vi "Go To Position.vi"(8 "error in (no error)":errorcluster, 9 "Target Position":T2, 10 "My Position":T2) -> (0 "error out":errorcluster, 1 "Arrived?":bool, 2 "Direction":T1)   [LabVIEW 2015, in "Common.lvlib"]
uses:
  Common.lvlib
  Position.ctl
  Type Defs/Direction Enum.ctl
  SubVIs/Read-Only Globals.vi
  SubVIs/Globals (private).vi
  Type Defs/SB Type Defs.lvlib
  Square/Square.lvclass
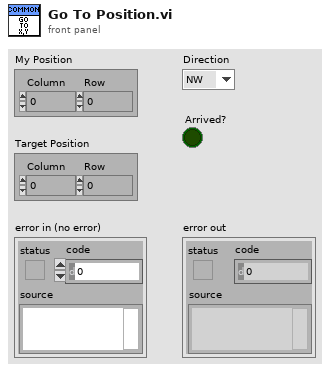
[diagram p1: front panel]
types:
  T1 = typedef "SB Type Defs.lvlib/Direction Enum.ctl" = enum16{"NW", "N", "NE", "E", "SE", "S", "SW", "W"}
  T2 = typedef "Common.lvlib/Position.ctl" = cluster{"Column":i32, "Row":i32}
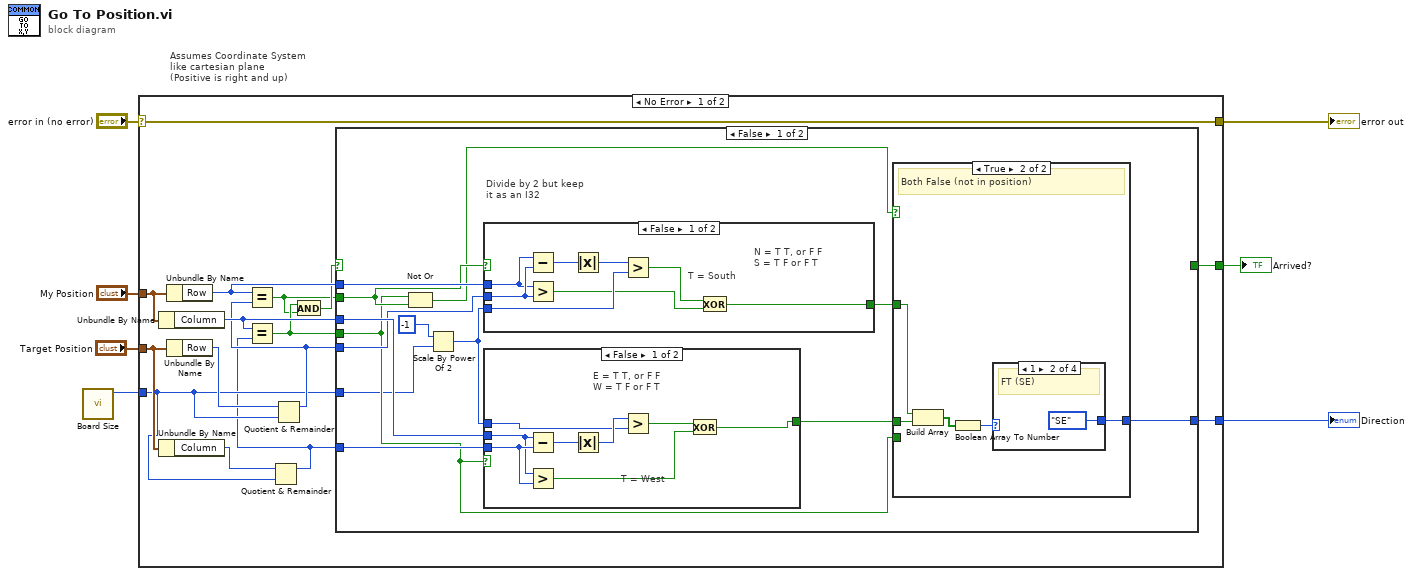
[diagram p0: block diagram]
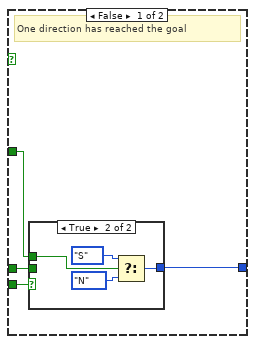
[diagram p2: hidden frame]
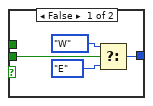
[diagram p3: hidden frame]
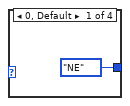
[diagram p4: hidden frame]
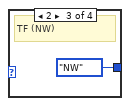
[diagram p5: hidden frame]
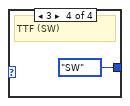
[diagram p6: hidden frame]
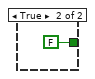
[diagram p7: hidden frame]
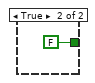
[diagram p8: hidden frame]
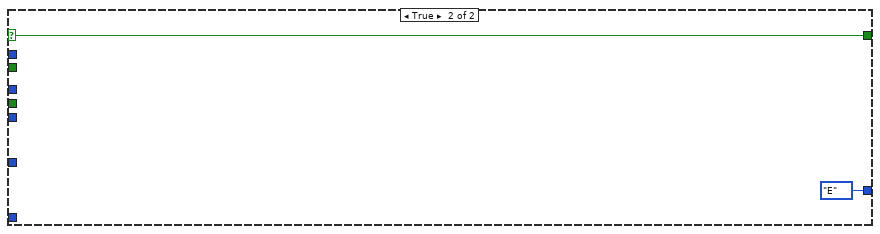
[diagram p9: hidden frame]
diagram:
  # "Assumes Coordinate System\nlike cartesian plane\n(Positive is right and up)"
  n1 = call "Board Size.vi"() -> ("Board Size"=w1:i32)  [unwired: 11 in]
  n2 = case shown="No Error" "error in (no error)" {
    selector: "error in (no error)" -> [w22 w77]
    tunnel: [w22 w77] -> w6
    tunnel: "Target Position" -> [w20 _]
    tunnel: "My Position" -> [w21 _]
    tunnel: [w16 _] -> w3
    tunnel: [w14 _] -> w2
    tunnel: w1 -> [w9 _]
    frame No Error {
      n3 = Unbundle By Name(w21) -> ("Column"=w19:i32)
      n4 = Unbundle By Name(w20) -> ("Column"=w10:i32)
      n5 = Unbundle By Name(w21) -> ("Row"=w18:i32)
      n6 = Unbundle By Name(w20) -> ("Row"=w12:i32)
      n7 = Quotient & Remainder(x=w10, y=w9) -> (x-y*floor(x/y)=w8:i32)  [unwired: 1 out]
      n8 = Equal?(x=w19, y=w8) -> (x = y?=w17:bool)
      n9 = Quotient & Remainder(x=w12, y=w9) -> (x-y*floor(x/y)=w11:i32)  [unwired: 1 out]
      n10 = Equal?(x=w18, y=w11) -> (x = y?=w13:bool)
      n11 = And(x=w17, y=w13) -> (x .and. y?=w15:bool)
      n12 = case shown="False" w15 {
        selector: w15 -> [_ w75]
        tunnel: w8 -> [w34 _]
        tunnel: w19 -> [w33 _]
        tunnel: w18 -> [w32 _]
        tunnel: w11 -> [w31 _]
        tunnel: w17 -> [w25 _]
        tunnel: [w24 Direction_Enum."E" ("Direction")] -> w16
        tunnel: [_ w75] -> w14
        tunnel: w13 -> [w29 _]
        tunnel: w9 -> [w23 _]
        frame False {
          # "Divide by 2 but keep it as an I32"
          n13 = Not Or(1:w29, 2:w25) -> (0:w28:bool)
          n14 = Scale By Power Of 2(n=i16 -1, x=w23) -> (x*2^n=w30:i32)
          n15 = case shown="False" w29 {
            tunnel: w30 -> [w62 _]
            tunnel: w31 -> [w61 _]
            tunnel: w32 -> [w60 _]
            tunnel: [w57 FALSE] -> w26
            frame False {
              # "T = South"
              # "N = T T, or F F\nS = T F or F T"
              n16 = Subtract(x=w60, y=w61) -> (x-y=w63:i32)
              n17 = Greater?(x=w60, y=w61) -> (0:w58:bool)
              n18 = Absolute Value(x=w63) -> (abs(x)=w64:i32)
              n19 = Greater?(x=w64, y=w62) -> (0:w59:bool)
              n20 = Exclusive Or(1:w58, 2:w59) -> (0:w57:bool)
            }
            frame True {
            }
          }
          n21 = case shown="False" w25 {
            tunnel: w30 -> [w71 _]
            tunnel: w34 -> [w70 _]
            tunnel: w33 -> [w69 _]
            tunnel: [w66 FALSE] -> w27
            frame False {
              # "T = West"
              # "E = T T, or F F\nW = T F or F T"
              n22 = Subtract(x=w69, y=w70) -> (x-y=w72:i32)
              n23 = Greater?(x=w69, y=w70) -> (0:w67:bool)
              n24 = Absolute Value(x=w72) -> (abs(x)=w73:i32)
              n25 = Greater?(x=w73, y=w71) -> (0:w68:bool)
              n26 = Exclusive Or(1:w67, 2:w68) -> (0:w66:bool)
            }
            frame True {
            }
          }
          n27 = case shown="True" w28 {
            tunnel: w27 -> [w38 w52]
            tunnel: w26 -> [w36 w51]
            tunnel: w25 -> [w39 _]
            tunnel: [w37 w48] -> w24
            frame False {
              # "One direction has reached the goal"
              n28 = case shown="True" w39 {
                tunnel: [w40 w44] -> w37
                tunnel: w38 -> [w43 _]
                tunnel: w36 -> [_ w45]
                frame False {
                  n29 = Select(t=Direction_Enum."W" ("Direction"), s=w43, f=Direction_Enum."E" ("Direction")) -> (s? t:f=w40:T1)
                }
                frame True {
                  n30 = Select(t=Direction_Enum."S" ("Direction"), s=w45, f=Direction_Enum."N" ("Direction")) -> (s? t:f=w44:T1)
                }
              }
            }
            frame True {
              # "Both False (not in position)"
              n31 = Build Array(w51, w52) -> (w50:bool[])
              n32 = Boolean Array To Number(Boolean array=w50) -> (number=w49:u32)
              n33 = case shown="1" w49 {
                tunnel: [Direction_Enum."NE" ("Direction") Direction_Enum."SE" ("Direction") Direction_Enum."NW" ("Direction") Direction_Enum."SW" ("Direction")] -> w48
                frame 0, Default {
                }
                frame 1 {
                  # "FT (SE)"
                }
                frame 2 {
                  # "TF (NW)"
                }
                frame 3 {
                  # "TTF (SW)"
                }
              }
            }
          }
        }
        frame True {
        }
      }
    }
    frame Error {
    }
  }
  "error out" <- w6
  "Direction" <- w3
  "Arrived?" <- w2
